vi "Error Query.vi"(8 "error in (no error)":errorcluster, 11 "VISA resource name":refnum<visa-resource-name>) -> (0 "error out":errorcluster, 1 "Error Message":string, 2 "Error Code":i32[](array[numeric]), 3 "VISA resource name out":refnum<visa-resource-name>)   [LabVIEW 2020, in "BK Precision 911X Series.lvlib"]
doc: "Queries the instrument for any errors in the instrument's error queue. It will continue to read errors until all errors have been read from the instrument. Any errors will be returned in the <B>error out</B> control.\n\n<B>Note:</B>\nThis VI is called automatically by most driver VIs so it is not usually necessary to call this in an application."
uses:
  BK Precision 911X Series.lvlib
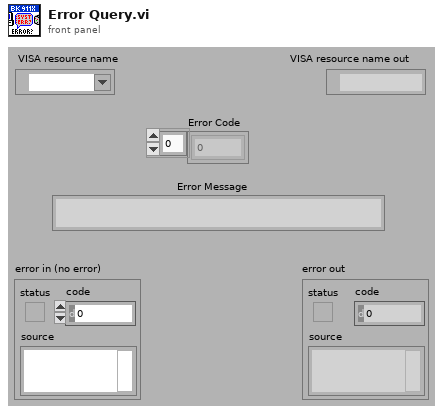
[diagram p1: front panel]
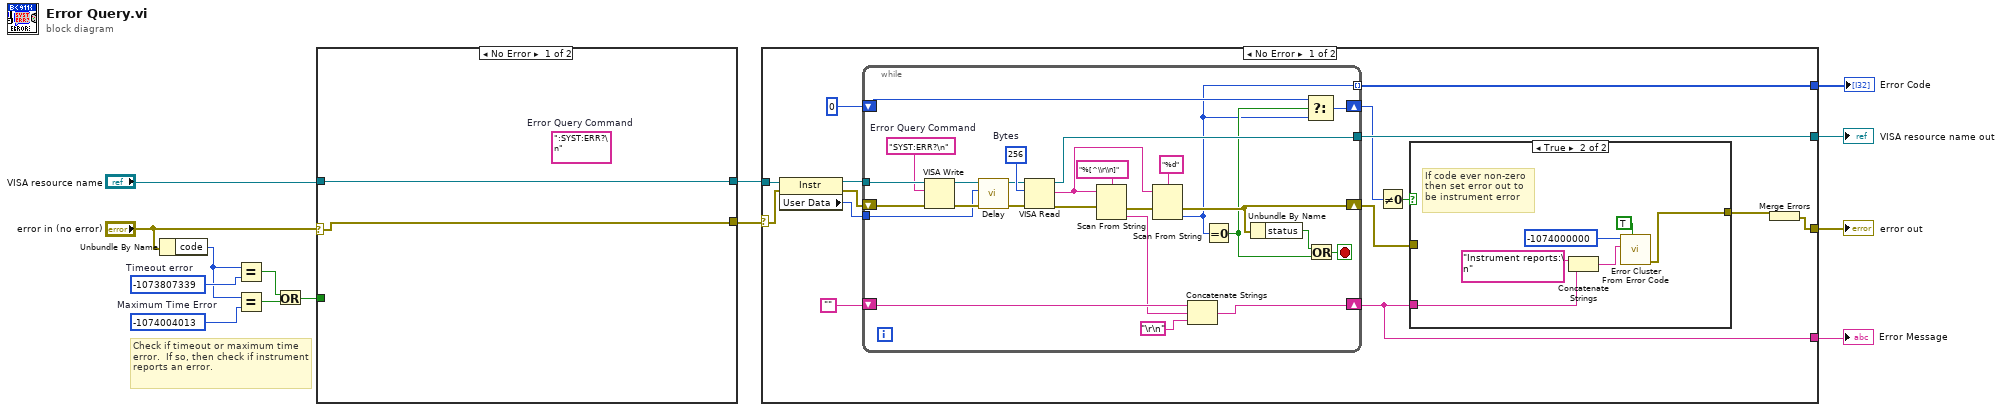
[diagram p0: block diagram]
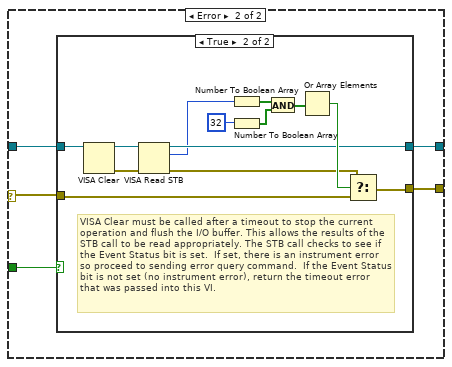
[diagram p2: hidden frame]
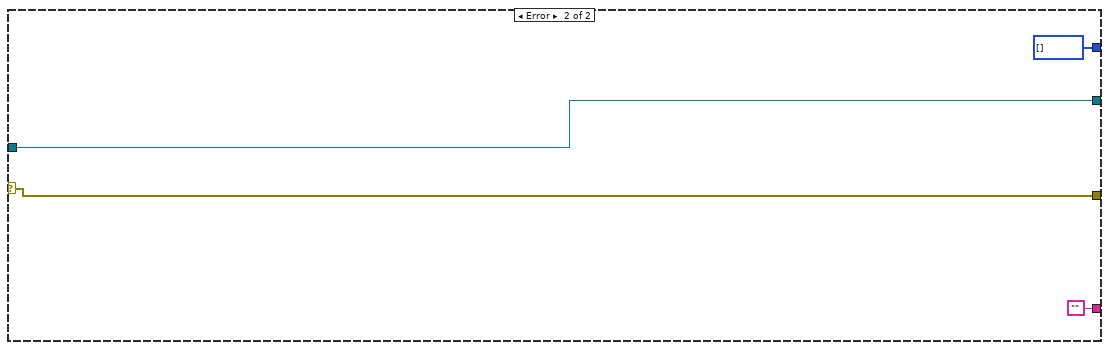
[diagram p5: hidden frame]
diagram:
  w5 = -1074004013  # Maximum Time Error
  w7 = -1073807339  # Timeout error
  # "Check if timeout or maximum time error.  If so, then check if instrument reports an error."
  n1 = Unbundle By Name("error in (no error)") -> ("code"=w6:i32)
  n2 = Equal?(x=w6, y=w7) -> (x = y?=w3:bool)
  n3 = Equal?(x=w6, y=w5) -> (x = y?=w4:bool)
  n4 = Or(x=w3, y=w4) -> (x .or. y?=w2:bool)
  n5 = case shown="No Error" "error in (no error)" {
    selector: "error in (no error)" -> [w15 w19]
    tunnel: "VISA resource name" -> [w16 w21]
    tunnel: [w16 w20] -> w9
    tunnel: [w15 w18] -> w10
    tunnel: w2 -> [_ w17]
    frame No Error {
      (unwired) ":SYST:ERR?\n"  # Error Query Command
    }
    frame Error {
      n6 = case shown="True" w17 {
        tunnel: w21 -> [w23 w29]
        tunnel: [w23 w26] -> w20
        tunnel: w19 -> [w22 w32]
        tunnel: [w22 w31] -> w18
        frame False {
          # "Error code not a timeout, so best to pass on to user."
        }
        frame True {
          # "VISA Clear must be called after a timeout to stop the current operation and flush the I/O buffer. This allows the results of the  STB call to be read appropriately. The STB call checks to see if the Event Status bit is set.  If set, there is an instrument error so proceed to sending error query command.  If the Event Status bit is not set (no instrument error), return the timeout error that was passed into this VI."
          n7 = VISA Clear(VISA resource name=w29) -> (VISA resource name out=w28:refnum<visa-resource-name>, error out=w27:errorcluster)  [unwired: 1 in]
          n8 = VISA Read STB(8:w27, 11:w28) -> (0:w25:errorcluster, 2:w24:u16, 3:w26:refnum<visa-resource-name>)
          n9 = Number To Boolean Array(number=w24) -> (Boolean array=w33:bool[])
          n10 = Number To Boolean Array(number=32) -> (Boolean array=w35:bool[])
          n11 = And(x=w33, y=w35) -> (x .and. y?=w34:bool[])
          n12 = Or Array Elements(Boolean array=w34) -> (logical OR=w30:bool)
          n13 = Select(t=w25, s=w30, f=w32) -> (s? t:f=w31:errorcluster)
        }
      }
    }
  }
  n14 = case shown="No Error" w10 {
    selector: w10 -> [w39 w85]
    tunnel: [w51 w88] -> w14
    tunnel: w9 -> [w41 w88]
    tunnel: [w49 w85] -> w13
    tunnel: [w44 ""] -> w12
    tunnel: [w43 i32[] []] -> w11
    frame No Error {
      n15 = property class="Instr"(reference=w41, error in=w39) -> (reference out=w40:refnum<visa-resource-name>, error out=w38:errorcluster, "User Data"=w37:u32)
      n16 = while {
        tunnel: [w84] -> w51
        tunnel: w40 -> [w83]
        shift-right: [w73] -> w44
        shift-left: "" -> [w76]
        shift-right: [w71] -> w45
        shift-left: 0 -> [w72]
        shift-right: [w69] -> w42
        shift-left: w38 -> [w70]
        tunnel: [w64] -> w43 mode=indexing
        tunnel: w37 -> [w59]
        stop <- w79 stop-if-true
        w82 = u32 256  # Bytes
        w81 = "SYST:ERR?\n"  # Error Query Command
        n17 = VISA Write(VISA resource name=w83, write buffer=w81, error in (no error)=w70) -> (VISA resource name out=w63:refnum<visa-resource-name>, error out=w62:errorcluster)  [unwired: 1 out]
        n18 = call "Delay.vi"("error in (no error)"=w62, "Delay Time (0 ms)"=w59, "VISA resource name"=w63) -> ("error out"=w61:errorcluster, "VISA resource name out"=w60:refnum<visa-resource-name>)  [unwired: 7 in]
        n19 = VISA Read(VISA resource name=w60, byte count=w82, error in (no error)=w61) -> (VISA resource name out=w84:refnum<visa-resource-name>, read buffer=w77:string, error out=w68:errorcluster)  [unwired: 1 out]
        n20 = Scan From String(format string="%[^\\r\\n]", input string=w77, error in=w68) -> (error out=w67:errorcluster, output 1=w74:string)  [unwired: 2 in, 2 out]
        n21 = Scan From String(format string="%d", input string=w77, error in=w67) -> (error out=w69:errorcluster, output 1=w64:i32)  [unwired: 2 in, 2 out]
        n22 = Concatenate Strings(w76, w74, "\r\n") -> (w73:string)
        n23 = Equal To 0?(x=w64) -> (x = 0?=w65:bool)
        n24 = Unbundle By Name(w69) -> ("status"=w66:bool)
        n25 = Select(t=w72, s=w65, f=w64) -> (s? t:f=w71:i32)
        n26 = Or(x=w66, y=w65) -> (x .or. y?=w79:bool)
      }
      n27 = Not Equal To 0?(x=w45) -> (x != 0?=w47:bool)
      n28 = case shown="True" w47 {
        tunnel: w44 -> [_ w57]
        tunnel: [w52 w53] -> w46
        tunnel: w42 -> [w52 _]
        frame False {
        }
        frame True {
          # "If code ever non-zero\nthen set error out to\nbe instrument error"
          n29 = Concatenate Strings("Instrument reports:\n" ("Source"), w57) -> (w54:string)
          n30 = call <vilib>:"Error Cluster From Error Code.vi"("show call chain? (False)"=TRUE, "error message (\"\")"=w54, "error code (0)"=-1074000000 ("Code")) -> ("error out"=w53:errorcluster)  [unwired: 6 in]
        }
      }
      n31 = Merge Errors(w46) -> (w49:errorcluster)
    }
    frame Error {
    }
  }
  "VISA resource name out" <- w14
  "error out" <- w13
  "Error Message" <- w12
  "Error Code" <- w11
